vi "Vision Processing.vi"() -> ()   [LabVIEW 2018]
doc: "This VI runs in parallel to other tasks. It gets images from the camera, processes them for color or shape and use that information to affect robot behavior."
uses:
  <vilib>/Rock Robotics/WPI/Camera/WPI_CameraImageSize.ctl
  <vilib>/Rock Robotics/WPI/Camera/WPI_CameraWhite Balance Values.ctl
  <vilib>/Rock Robotics/WPI/Camera/WPI_CameraExposure Values.ctl
  <vilib>/Rock Robotics/WPI/Camera/WPI_CameraFrameRate.ctl
  Robot Global Data.vi
  <vilib>/vision/NI_Vision_Development_Module.lvlib
panel:
  in  "Image Size 2":T1=enum."160x120"
  in  "error in (no error) 2":errorcluster
  in  "Hue":cluster{"Lower value":i32, "Upper value":i32}={"Lower value"=80, "Upper value"=130}
  in  "Sat":cluster{"Lower value":i32, "Upper value":i32}={"Lower value"=130, "Upper value"=255}
  in  "Lum":cluster{"Lower value":i32, "Upper value":i32}={"Lower value"=30, "Upper value"=100}
  out "Map":T2
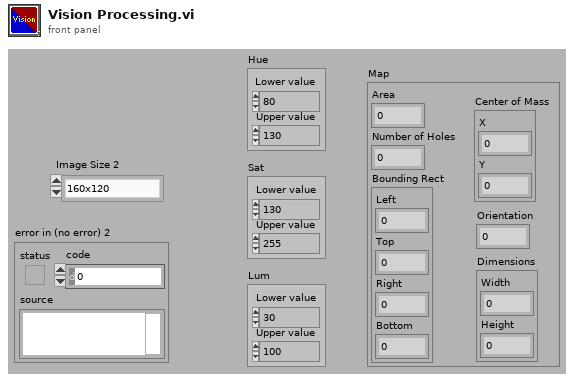
[diagram p1: front panel]
types:
  T1 = typedef "WPI_CameraImageSize.ctl" = enum16{"640x480", "320x240", "160x120", "Custom"}
  T2 = cluster{"Area":dbl, "Number of Holes":dbl, "Bounding Rect":cluster{"Left":dbl, "Top":dbl, "Right":dbl, "Bottom":dbl}, "Center of Mass":cluster{"X":dbl, "Y":dbl}, "Orientation":dbl, "Dimensions":cluster{"Width":dbl, "Height":dbl}}
  T3 = typedef "Image Type" = u32
  T4 = typedef "WPI_CameraFrameRate.ctl" = u32
  T5 = typedef "WPI_CameraExposure Values.ctl" = enum16{"Auto", "Flicker-free 50 Hz", "Flicker-free 60 Hz", "Hold current", "Custom"}
  T6 = typedef "WPI_CameraWhite Balance Values.ctl" = enum16{"Auto", "Fixed indoor", "Fixed outdoor 1", "Fixed outdoor 2", "Fixed fluorescent 1", "Fixed fluorescent 2", "Hold current", "Custom"}
  T7 = typedef "WPI_CameraDevRef.ctl" = cluster{"Camera Address":string, "CameraStatus":errorcluster}
  T8 = typedef "IMAQ Image.ctl" = refnum<image>
  T9 = typedef "Particle Parameters" = i32
  T10 = cluster{"Measurement Parameter":T9, "Range Lower Value":dbl, "Range Upper Value":dbl, "Range":bool, "Measurement Type":bool}[]
  T11 = cluster{"Area":dbl, "Number of Holes":dbl, "Bounding Rect":cluster{"Left":dbl, "Top":dbl, "Right":dbl, "Bottom":dbl}, "Center of Mass":cluster{"X":dbl, "Y":dbl}, "Orientation":dbl, "Dimensions":cluster{"Width":dbl, "Height":dbl}}[]
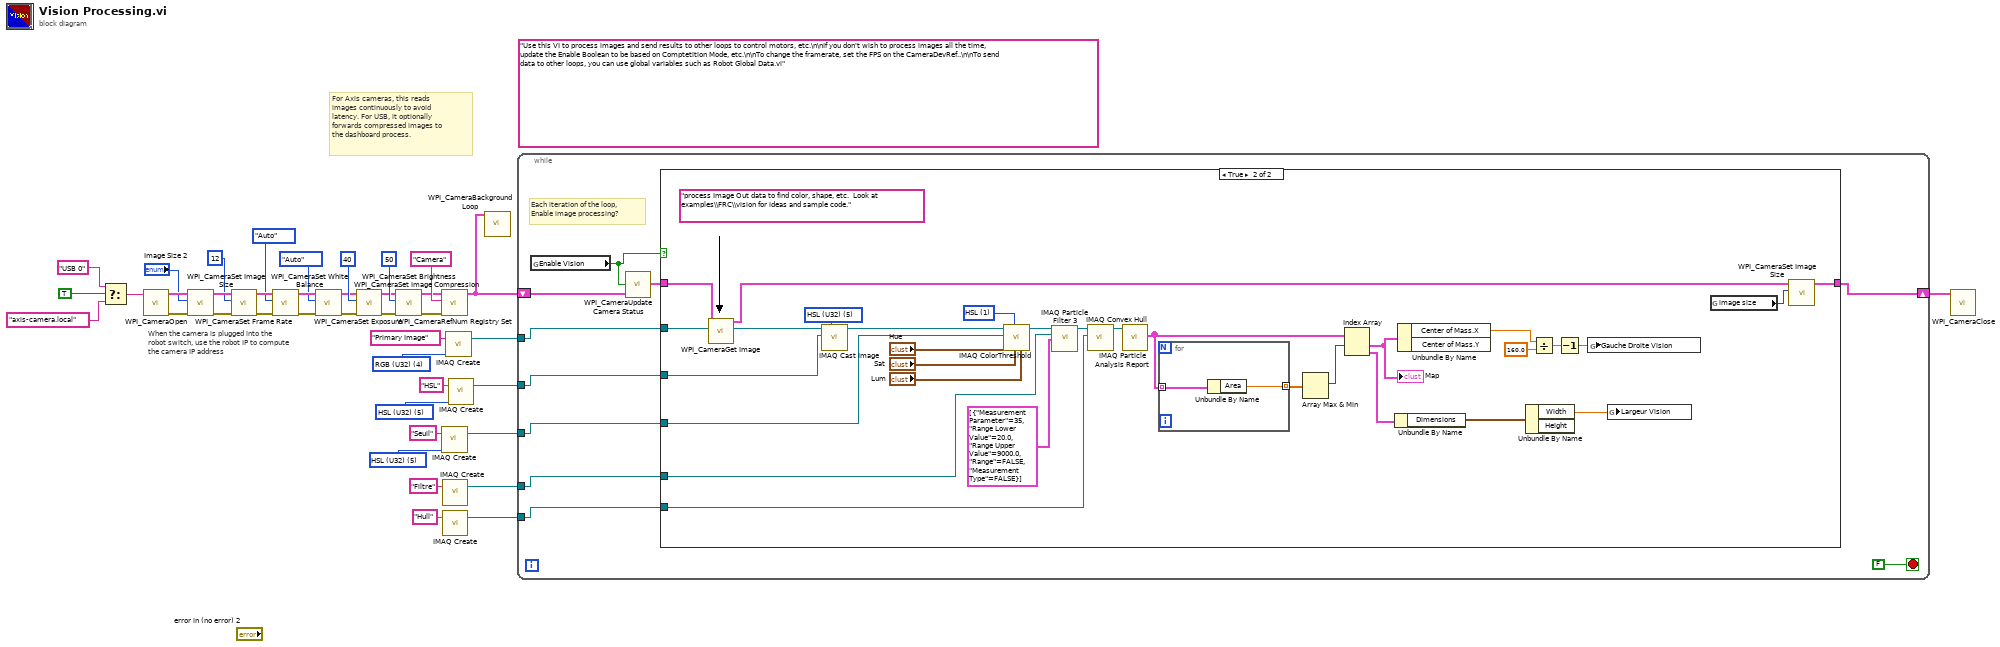
[diagram p0: block diagram]
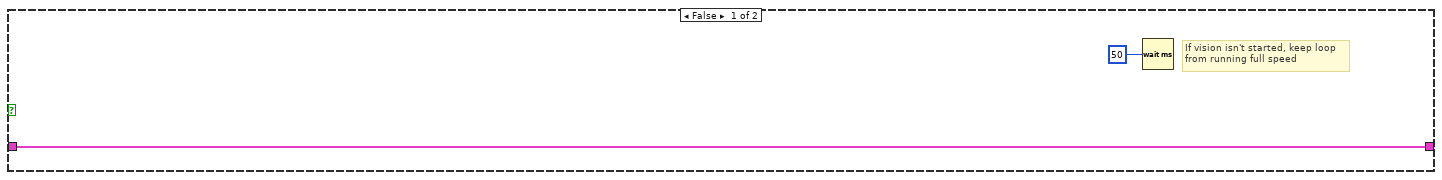
[diagram p2: hidden frame]
diagram:
  w7 = T3 5 items=["Grayscale (U8)", "Grayscale (I16)", "Grayscale (SGL)", "Complex (CSG)", "RGB (U32)", "HSL (U32)", "RGB (U64)"] ("Image Type")
  w9 = T3 5 items=["Grayscale (U8)", "Grayscale (I16)", "Grayscale (SGL)", "Complex (CSG)", "RGB (U32)", "HSL (U32)", "RGB (U64)"] ("Image Type")
  (unwired) "Use this VI to process images and send results to other loops to control motors, etc.\n\nIf you don't wish to process images all the time, update the Enable Boolean to be based on Comptetition Mode, etc.\n\nTo change the framerate, set the FPS on the CameraDevRef..\n\nTo send data to other loops, you can use global variables such as Robot Global Data.vi"
  w40 = T3 4 items=["Grayscale (U8)", "Grayscale (I16)", "Grayscale (SGL)", "Complex (CSG)", "RGB (U32)", "HSL (U32)", "RGB (U64)"] ("Image Type")
  # "When the camera is plugged into the\nrobot switch, use the robot IP to compute\nthe camera IP address"
  # "For Axis cameras, this reads\nimages continuously to avoid\nlatency. For USB, it optionally\nforwards compressed images to\nthe dashboard process."
  n1 = Select(t="USB 0" ("format string"), s=TRUE ("dot notation? (F)"), f="axis-camera.local" ("format string")) -> (s? t:f=w12:string)
  n2 = call <vilib>:"WPI_CameraOpen.vi"("Camera Address"=w12) -> ("error out"=w28:errorcluster, "CameraDevRef"=w29:T7)  [unwired: 1 in, 8 out]
  n3 = call <vilib>:"WPI_CameraSet Image Size.vi"("error in (no error)"=w28, "Image Size"="Image Size 2", "CameraDevRef"=w29) -> ("error out"=w27:errorcluster, "CameraDevRef Out"=w30:T7)  [unwired: 1 in, 6 out]
  n4 = call <vilib>:"WPI_CameraSet Frame Rate.vi"("error in (no error)"=w27, "Frame Rate (fps)"=T4 12, "CameraDevRef"=w30) -> ("error out"=w26:errorcluster, "CameraDevRef Out"=w32:T7)  [unwired: 7 out]
  n5 = call <vilib>:"WPI_CameraSet White Balance.vi"("error in (no error)"=w26, "White Balance"=WPI_CameraWhite_Balance_Values."Auto", "CameraDevRef"=w32) -> ("error out"=w25:errorcluster, "CameraDevRef Out"=w31:T7)  [unwired: 1 in, 6 out]
  n6 = call <vilib>:"WPI_CameraSet Exposure.vi"("error in (no error)"=w25, "Exposure"=WPI_CameraExposure_Values."Auto", "CameraDevRef"=w31) -> ("error out"=w24:errorcluster, "CameraDevRef Out"=w34:T7)  [unwired: 1 in, 6 out]
  n7 = call <vilib>:"WPI_CameraSet Image Compression.vi"("error in (no error)"=w24, "Compression"=40, "CameraDevRef"=w34) -> ("error out"=w23:errorcluster, "CameraDevRef Out"=w33:T7)  [unwired: 7 out]
  n8 = call <vilib>:"WPI_CameraSet Brightness.vi"("error in (no error)"=w23, "Brightness"=50, "CameraDevRef"=w33) -> ("error out"=w21:errorcluster, "CameraDevRef Out"=w22:T7)  [unwired: 1 in, 6 out]
  n9 = call <vilib>:"WPI_CameraRefNum Registry Set.vi"("error in (no error)"=w21, "refnum name"="Camera", "CameraDevRef"=w22) -> ("CameraDevRef"=w17:T7)  [unwired: 1 in, 7 out]
  n10 = call "IMAQ Create"("Image Name"="Seuil", "Image Type"=w7) -> ("New Image"=w5:T8)  [unwired: 2 in, 2 out]
  n11 = call "IMAQ Create"("Image Name"="Filtre") -> ("New Image"=w3:T8)  [unwired: 3 in, 2 out]
  n12 = call "IMAQ Create"("Image Name"="Hull") -> ("New Image"=w1:T8)  [unwired: 3 in, 2 out]
  n13 = call "IMAQ Create"("Image Name"="Primary Image", "Image Type"=w40) -> ("New Image"=w38:T8)  [unwired: 2 in, 2 out]
  n14 = call "IMAQ Create"("Image Name"="HSL", "Image Type"=w9) -> ("New Image"=w8:T8)  [unwired: 2 in, 2 out]
  n15 = call <vilib>:"WPI_CameraBackground Loop.vi"("CameraDevRef"=w17) -> ()  [unwired: 11 in]
  n16 = while {
    shift-right: [w49] -> w15
    shift-left: w17 -> [w47]
    tunnel: w38 -> [w48]
    tunnel: w8 -> [w45]
    tunnel: w5 -> [w44]
    tunnel: w3 -> [w43]
    tunnel: w1 -> [w42]
    stop <- FALSE stop-if-true
    # "Each iteration of the loop,\nEnable image processing?"
    n17 = global read "Robot Global Data.vi" "Enable Vision"() -> (w41:bool)
    n18 = call <vilib>:"WPI_CameraUpdate Camera Status.vi"("CameraDevRef In"=w47, "Enable Vision"=w41) -> ("CameraDevRef Out"=w46:T7)  [unwired: 3 in]
    n19 = case shown="True" w41 {
      tunnel: w48 -> [_ w82]
      tunnel: [w52 w83] -> w49
      tunnel: w46 -> [w52 w61]
      tunnel: w45 -> [_ w65]
      tunnel: w44 -> [_ w64]
      tunnel: w43 -> [_ w62]
      tunnel: w42 -> [_ w63]
      frame False {
        # "If vision isn't started, keep loop\nfrom running full speed"
        n20 = Wait (ms)(milliseconds to wait=u32 50) -> ()  [unwired: 1 out]
      }
      frame True {
        w79 = u16 1 items=["RGB", "HSL", "HSV", "HSI"] ("Color Mode")
        w80 = T3 5 items=["Grayscale (U8)", "Grayscale (I16)", "Grayscale (SGL)", "Complex (CSG)", "RGB (U32)", "HSL (U32)", "RGB (U64)", "Grayscale (U16)"] ("Image Type")
        (unwired) "process Image Out data to find color, shape, etc.  Look at examples\\FRC\\vision for ideas and sample code."
        n21 = call <vilib>:"WPI_CameraGet Image.vi"("Image"=w82, "CameraDevRef"=w61) -> ("Image Out"=w66:T8, "CameraDevRef Out"=w60:T7)  [unwired: 1 in, 7 out]
        n22 = call "IMAQ Cast Image"("Image Type"=w80, "Image Dst"=w65, "Image Src"=w66) -> ("Image Dst Out"=w70:T8)  [unwired: 7 in, 1 out]
        n23 = call "IMAQ ColorThreshold"("Blue or Luma or Val or Inten Range"="Lum", "Green or Sat Range"="Sat", "Color Mode"=w79, "Red or Hue Range"="Hue", "Image Dst"=w64, "Image Src"=w70) -> ("Image Dst Out"=w75:T8)  [unwired: 4 in, 1 out]
        n24 = call "IMAQ Particle Filter 3"("Image Src"=w75, "Image Dst"=w62, "Selection Values"=T10 [{"Measurement Parameter"=35, "Range Lower Value"=20.0, "Range Upper Value"=9000.0, "Range"=FALSE, "Measurement Type"=FALSE}]) -> ("Image Dst Out"=w71:T8)  [unwired: 10 in, 2 out]
        n25 = call "IMAQ Convex Hull"("Image Dst"=w63, "Image Src"=w71) -> ("Image Dst Out"=w73:T8)  [unwired: 8 in, 1 out]
        n26 = call "IMAQ Particle Analysis Report"("Image"=w73) -> ("Particle Reports (Pixels)"=w68:T11)  [unwired: 5 in, 5 out]
        n27 = for {
          tunnel: w68 -> [w85] mode=indexing
          tunnel: [w84] -> w69 mode=indexing
          n28 = Unbundle By Name(w85) -> ("Area"=w84:dbl)
        }
        n29 = Array Max & Min(array=w69) -> (max index (indices)=w67:i32)  [unwired: 3 out]
        n30 = Index Array(array=w68, index #1=w67) -> (element #1=w72:T2, element #2=w59:T2)  [unwired: 1 in]
        "Map" <- w72
        n31 = Unbundle By Name(w59) -> ("Dimensions"=w58:cluster{"Width":dbl, "Height":dbl})
        n32 = Unbundle By Name(w72) -> ("Center of Mass.X"=w56:dbl)  [unwired: 1 out]
        n33 = Unbundle By Name(w58) -> ("Width"=w57:dbl)  [unwired: 1 out]
        n34 = Divide(x=w56, y=160.0) -> (x/y=w54:dbl)
        n35 = Decrement(x=w54) -> (x-1=w53:dbl)
        n36 = global write "Robot Global Data.vi" "Gauche Droite Vision"(w53) -> ()
        n37 = global write "Robot Global Data.vi" "Largeur Vision"(w57) -> ()
        n38 = global read "Robot Global Data.vi" "image size"() -> (w81:T1)
        n39 = call <vilib>:"WPI_CameraSet Image Size.vi"("Image Size"=w81, "CameraDevRef"=w60) -> ("CameraDevRef Out"=w83:T7)  [unwired: 2 in, 7 out]
      }
    }
  }
  n40 = call <vilib>:"WPI_CameraClose.vi"("CameraDevRef"=w15) -> ()  [unwired: 1 in, 10 out]
